vi "ExFFAccumCirBufBin2x.vi"() -> ()   [LabVIEW 2010]
panel:
  out "Paired mode":bool
  out "Accum mode":bool
  out "FF Available?":bool
  in  "Accum Mode":bool
  in  "Accum Number":u32
  out "Accum Number":u32
  in  "Exposure":dbl min=0.0 step=1e-06 format="%.6f"
  in  "stop":bool
  in  "Store":bool
  out "error out":errorcluster
  in  "error in (no error)":errorcluster
  # "ExFFAccumCirBufBin2x.vi:\nThis example shows how the Accum\nmode works on a CoolSnap Hq with \nDIF works. It disables the paired mode\nsince it doesn't work at the same time\nas Accum mode."
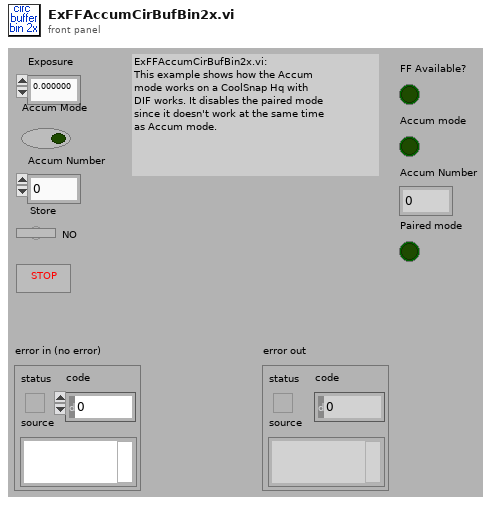
[diagram p1: front panel]
types:
  T1 = cluster{"acquire focus mode":u32, "Exposure":dbl, "Number of Images":u32, "Software accumulation":u32}
  T2 = cluster{"Camera Handle":u32, "Pulser Handle":u32, "File Handle":u32, "Display Handle":u32, "Image Handle":u32}
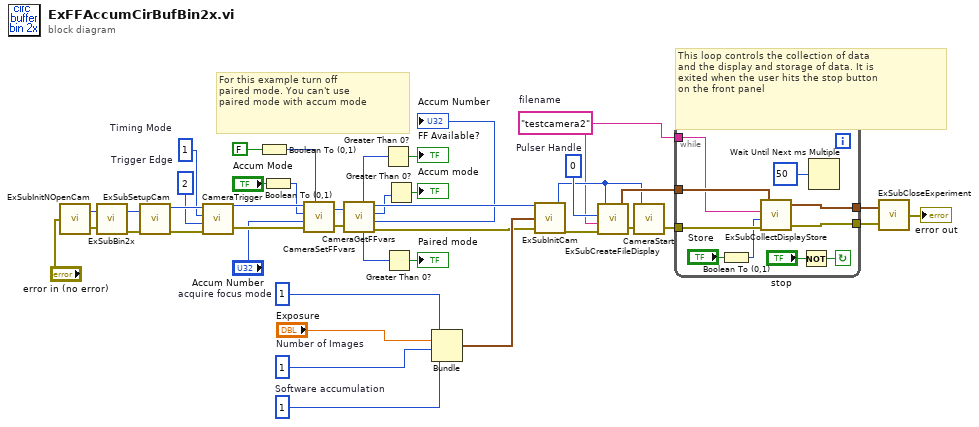
[diagram p0: block diagram]
diagram:
  w23 = u32 0  # Pulser Handle
  w24 = u32 1  # Timing Mode
  w25 = u32 2  # Trigger Edge
  w28 = u32 1  # acquire focus mode
  w27 = u32 1  # Number of Images
  w26 = u32 1  # Software accumulation
  w9 = "testcamera2"  # filename
  # "This loop controls the collection of data\nand the display and storage of data. It is \nexited when the user hits the stop button \non the front panel"
  # "For this example turn off\npaired mode. You can't use\npaired mode with accum mode"
  n1 = call "ExSubInitNOpenCam.vi"("error in (no error)"="error in (no error)") -> ("Camera Handle"=w30:u32, "error out"=w29:errorcluster)
  n2 = call "ExSubBin2x.vi"("error in (no error)"=w29, "Camera Handle"=w30) -> ("error out"=w21:errorcluster, "Camera Handle"=w20:u32)
  n3 = call "ExSubSetupCam.vi"("error in (no error)"=w21, "Camera Handle"=w20) -> ("error out"=w33:errorcluster, "Camera Handle"=w34:u32)
  n4 = call <userlib>:"CameraTrigger.vi"("error in"=w33, "Trigger Edge"=w25, "Timing Mode"=w24, "Camera Handle"=w34) -> ("error out"=w14:errorcluster, "Camera Handle"=w13:u32)
  n5 = Boolean To (0,1)(Boolean=FALSE) -> (0, 1=w12:i16)
  n6 = Boolean To (0,1)(Boolean="Accum Mode") -> (0, 1=w8:i16)
  n7 = call <userlib>:"CameraSetFFvars.vi"(0:w13, 1:w8, 2:"Accum Number", 3:w14, 4:w12) -> (5:w16:u32, 6:w15:errorcluster)
  n8 = call <userlib>:"CameraGetFFvars.vi"(0:w16, 1:w15) -> (2:w2:u8, 3:w3:u32, 4:w19:u32, 5:w1:u32, 6:→"Accum Number":u32, 7:w18:errorcluster)
  n9 = Greater Than 0?(x=w2) -> (x > 0?=→"FF Available?":bool)
  n10 = Greater Than 0?(x=w3) -> (x > 0?=→"Paired mode":bool)
  n11 = Greater Than 0?(x=w1) -> (x > 0?=→"Accum mode":bool)
  n12 = Bundle("acquire focus mode"=w28, "Exposure"="Exposure", "Number of Images"=w27, "Software accumulation"=w26) -> (w40:T1)  [unwired: 1 in]
  n13 = call "ExSubInitCam.vi"("error in (no error)"=w18, "Camera Information"=w40, "Camera Handle"=w19) -> ("error out"=w39:errorcluster, "Camera Handle"=w22:u32)
  n14 = call "ExSubCreateFileDisplay.vi"("error in (no error)"=w39, "File and Display Name"=w9, "Pulser Handle"=w23, "Camera Handle"=w22) -> ("error out"=w31:errorcluster, "Handles Out"=w38:T2)
  n15 = call <userlib>:"CameraStart.vi"("error in"=w31, "Camera Handle"=w22) -> ("error out"=w32:errorcluster)  [unwired: 1 out]
  n16 = while {
    tunnel: w38 -> [w51]
    tunnel: w32 -> [w50]
    tunnel: w9 -> [w43]
    tunnel: [w48] -> w36
    tunnel: [w49] -> w37
    stop <- w46 continue-if-true
    n17 = Boolean To (0,1)(Boolean="Store") -> (0, 1=w44:i16)
    n18 = call "ExSubCollectDisplayStore.vi"("error in (no error)"=w50, "Store flag"=w44, "Display Title"=w43, "Handle Cluster"=w51) -> ("error out"=w48:errorcluster, "Handle Cluster Out"=w49:T2)  [unwired: 1 out]
    n19 = Not(x="stop") -> (.not. x?=w46:bool)
    n20 = Wait Until Next ms Multiple(millisecond multiple=u32 50) -> ()  [unwired: 1 out]
  }
  n21 = call "ExSubCloseExperiment.vi"("error in (no error)"=w36, "Handles In"=w37) -> ("error out"=→"error out":errorcluster)
